vi "Barrier Init.vi"(8 "error in (no error)":errorcluster, 9 "count":u32, 10 "Barrier Attr in":T2, 11 "Barrier in":T1) -> (0 "error out":errorcluster, 2 "Barrier Attr out":T2, 3 "Barrier out":T1)   [LabVIEW 2013, in "Linux RT IPC.POSIX Threads.lvlib" / "Barrier.lvclass"]
doc: "Calls pthread_barrier_init() on the pthread barrier object encapsulated by Barrier.\n\nThis VI initializes the barrier object and sets its attributes using the attributes contained in the Barrier Attr object.\n\nRefer to online POSIX documentation for more information."
uses:
  Barrier.lvclass
  Controls/reference.ctl
  Barrier Attr/Controls/reference.ctl
  Barrier Attr/Barrier Attr.lvclass
  POSIX Thread Object/POSIX Thread Object.lvclass/POSIX Thread Object.ctl
  POSIX Thread Object/Private VIs/libpthread path.vi
  POSIX Thread Object/Private VIs/get pthread error.vi
  POSIX Thread Object/POSIX Thread Object.lvclass
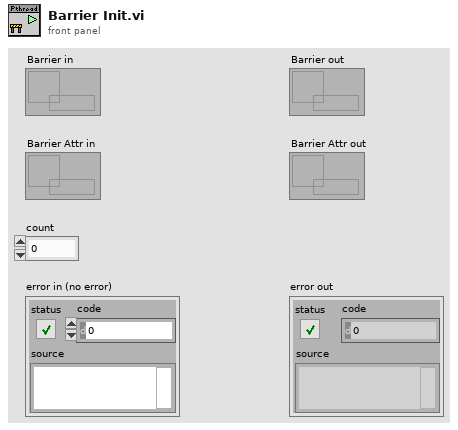
[diagram p1: front panel]
types:
  T1 = typedef "Linux RT IPC.POSIX Threads.lvlib/Barrier.lvclass/reference.ctl" = refnum<data-value>
  T2 = typedef "Linux RT IPC.POSIX Threads.lvlib/Barrier Attr.lvclass/reference.ctl" = refnum<data-value>
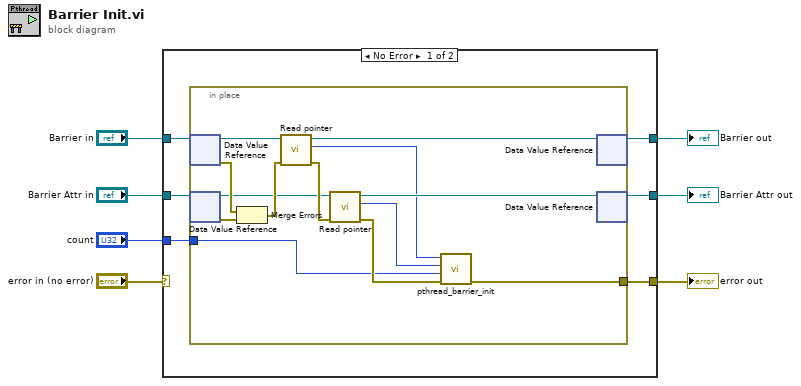
[diagram p0: block diagram]
diagram:
  n1 = case shown="No Error" "error in (no error)" {
    selector: "error in (no error)" -> [_ w29]
    tunnel: [w11 w29] -> w7
    tunnel: [w13 w28] -> w6
    tunnel: [w12 w27] -> w5
    tunnel: "Barrier Attr in" -> [w10 w27]
    tunnel: "Barrier in" -> [w9 w28]
    tunnel: "count" -> [w8 _]
    frame No Error {
      n2 = in-place {
        in-place-border: [w18] -> w11
        in-place-border: w8 -> [w14]
        n3 = in-place-dvr #1(w9) -> (w26:refnum<class "Barrier.lvclass">, w23:errorcluster)
        n4 = in-place-dvr #2(w10) -> (w19:refnum<class "Barrier Attr.lvclass">, w24:errorcluster)
        n5 = Merge Errors(w23, w24) -> (w22:errorcluster)
        n6 = call "Read pointer.vi"("error in (no error)"=w22, "POSIX Thread Object in"=w26) -> ("error out"=w21:errorcluster, "pointer"=w15:u64, "POSIX Thread Object out"=w25:refnum<class "Barrier.lvclass">)  [unwired: 7 in]
        n7 = call "Read pointer.vi"("error in (no error)"=w21, "POSIX Thread Object in"=w19) -> ("error out"=w17:errorcluster, "pointer"=w16:u64, "POSIX Thread Object out"=w20:refnum<class "Barrier Attr.lvclass">)  [unwired: 7 in]
        n8 = call "pthread_barrier_init.vi"("error in (no error)"=w17, "count"=w14, "barrier attr ptr in"=w16, "barrier ptr in"=w15) -> ("error out"=w18:errorcluster)  [unwired: 5 in, 2 out]
        n9 = in-place-dvr #1(w25) -> (w13:T1)  [unwired: 1 out]
        n10 = in-place-dvr #2(w20) -> (w12:T2)  [unwired: 1 out]
      }
    }
    frame Error {
    }
  }
  "Barrier out" <- w6
  "error out" <- w7
  "Barrier Attr out" <- w5
